vi "UV-VIS SetMultiTrack.vi"(0 "Control in":refnum<class "UV-VIS.lvclass">, 1 "height":i32, 2 "offset":i32, 3 "error in (no error)":errorcluster, 4 "number":i32) -> (5 "bottom":i32, 6 "Control out":refnum<class "UV-VIS.lvclass">, 7 "DLL error code":u32, 8 "gap":i32, 9 "error out":errorcluster)   [LabVIEW 2015, in "UV-VIS.lvclass"]
doc: "This function will set the multi-track parameters. The tracks are automatically spread evenly over the detector. Validation of the parameters is carried out in the following order: number of tracks, track height and the offset. The first pixels row of the first track is returned via ‘bottom’. The number of rows between each track is returned via ‘gap’.\n\n<B>Parameters:</B>\nnumber - number tracks\n Valid values 1 to number of vertical pixels\nheight - height of each track\n Valid values >0 (maximum depends on number of tracks)\noffset - vertical displacement of tracks\n Valid values depend on number of tracks and track height\nbottom - first pixels row of the first track\ngap - number of rows between each track (could be 0)\n\n<B>Error codes:</B>\nDRV_SUCCESS - Parameters set.\nDRV_NOT_INITIALIZED - System not initialized.\nDRV_ACQUIRING - Acquisition in progress.\nDRV_P1INVALID - Number of tracks invalid.\nDRV_P2INVALID - Track height invalid.\nDRV_P3INVALID - Offset invalid.\n\n<B>NOTES:</B>\n<B>NOT available on iXon.</B>"
uses:
  UV-VIS.lvclass
  Detector.lvclass/Detector.ctl
  Detector.lvclass
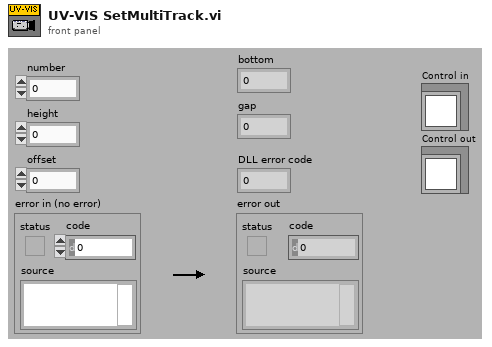
[diagram p1: front panel]
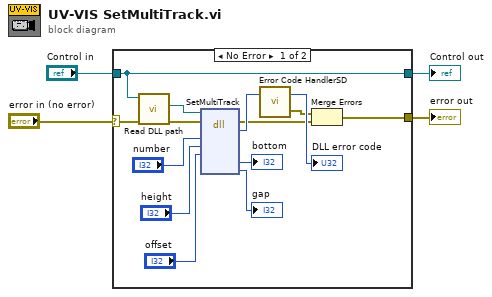
[diagram p0: block diagram]
diagram:
  n1 = case shown="No Error" "error in (no error)" {
    selector: "error in (no error)" -> [w10 w20]
    tunnel: [w5 w20] -> w3
    tunnel: [w11 w19] -> w2
    tunnel: "Control in" -> [w11 w19]
    frame No Error {
      n2 = call "Read DLL path.vi"("error in (no error)"=w10, "Detector in"=w11) -> ("error out"=w9:errorcluster, "DLL path"=w8:path)  [unwired: 7 in, 1 out]
      n3 = dll-call lib="S:/TRANCON/DLL/Atmcd32d.dll" fn="SetMultiTrack"(path in=w8, error in=w9, "number"="number", "height"="height", "offset"="offset") -> (error out=w7:errorcluster, "return type"=w18:u32, "bottom"=→"bottom":i32, "gap"=→"gap":i32)  [unwired: 6 in, 1 out]
      n4 = call "Error Code HandlerSD.vi"("DLL error code"=w18) -> ("error out"=w6:errorcluster, "dup DLL error code"=→"DLL error code":u32)  [unwired: 1 in]
      n5 = Merge Errors(w6, w7) -> (w5:errorcluster)
    }
    frame Error {
    }
  }
  "error out" <- w3
  "Control out" <- w2
